vi "Filter Items by Name.vi"(8 "error in (no error)":errorcluster, 9 "Target Names in":string[](array[string]), 10 "Build Specifications in":string[](array[string]), 11 "CD Build Tools in":refnum<class "Project Build Tools.lvclass">) -> (0 "error out":errorcluster, 1 "Target Names out":string[](array[string]), 2 "Build Specifications out":string[](array[string]), 3 "CD Build Tools out":refnum<class "Project Build Tools.lvclass">)   [LabVIEW 2019, in "Project Build Tools.lvclass"]
uses:
  Project Build Tools.lvclass
  Project Build Tools.lvclass/Project Build Tools.ctl
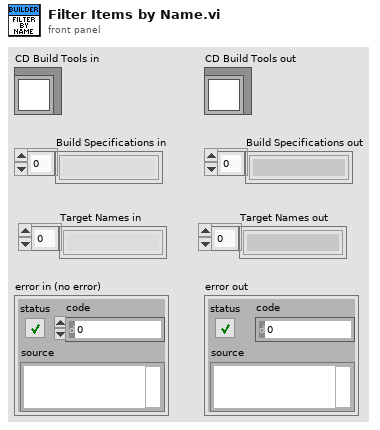
[diagram p1: front panel]
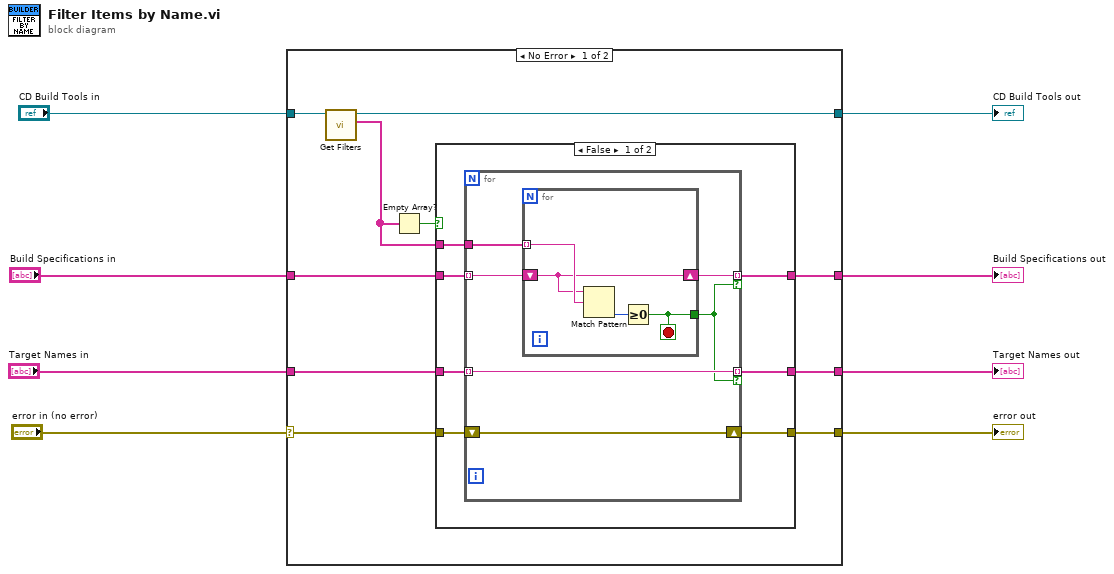
[diagram p0: block diagram]
diagram:
  n1 = case shown="No Error" "error in (no error)" {
    selector: "error in (no error)" -> [w13 w39]
    tunnel: [w18 _] -> w8
    tunnel: "Build Specifications in" -> [w17 _]
    tunnel: [w16 w40] -> w6
    tunnel: "CD Build Tools in" -> [w15 w40]
    tunnel: [w14 w39] -> w4
    tunnel: "Target Names in" -> [w10 _]
    tunnel: [w9 _] -> w1
    frame No Error {
      n2 = call "Get Filters.vi"("CD Build Tools in"=w15) -> ("Filters"=w12:string[], "CD Build Tools out"=w16:refnum<class "Project Build Tools.lvclass">)  [unwired: 9 in]
      n3 = Empty Array?(array=w12) -> (empty?=w11:bool)
      n4 = case shown="False" w11 {
        tunnel: [w25 w38] -> w18
        tunnel: w12 -> [w24 _]
        tunnel: w17 -> [w23 w38]
        tunnel: [w22 w37] -> w14
        tunnel: w13 -> [w21 w37]
        tunnel: w10 -> [w20 w36]
        tunnel: [w19 w36] -> w9
        frame False {
          n5 = for {
            tunnel: w23 -> [w30] mode=indexing
            tunnel: w24 -> [w31]
            tunnel: [w29] -> w25 mode=indexing if=w26
            shift-right: [w28] -> w22
            shift-left: w21 -> [w28]
            tunnel: w20 -> [w27] mode=indexing
            tunnel: [w27] -> w19 mode=indexing if=w26
            n6 = for {
              tunnel: w31 -> [w35] mode=indexing
              shift-right: [w33] -> w29
              shift-left: w30 -> [w33]
              tunnel: [w32] -> w26
              stop <- w32 stop-if-true
              n7 = Match Pattern(string=w33, regular expression=w35) -> (offset past match=w34:i32)  [unwired: 1 in, 3 out]
              n8 = Greater Or Equal To 0?(x=w34) -> (x >= 0?=w32:bool)
            }
          }
        }
        frame True {
        }
      }
    }
    frame Error {
    }
  }
  "error out" <- w4
  "Build Specifications out" <- w8
  "CD Build Tools out" <- w6
  "Target Names out" <- w1
